vi "Powerlawfit_Ranjani.vi"() -> ()   [LabVIEW 2020]
uses:
  <vilib>/Analysis/NI_AALPro.lvlib
panel:
  in  "parameter bounds":T1={"amp min"=-inf, "amp max"=inf, "power min"=-inf, "power max"=inf, "offset min"=-0.0001, "offset max"=0.0001}
  out "residue":dbl=1.2236868285246925e-12
  out "amplitude":dbl=1.9889547263019e-06
  out "Fitoffset":dbl=1.9090068470777766e-05
  out "power":dbl=2.2722781909445917
  in  "Tab Control":enum32{"Drag R and 4T R", " Line cut"}(tab)=enum." Line cut"
  in  "Input figure":cluster{dbl[], dbl[]}[](graph)
  out "Mean vs Curve":cluster{dbl[], dbl[]}(graph)
  in  "Group #":i32=40
  out "Power vs Cursorx":cluster{dbl[], dbl[]}(graph)
  out "Waveform Chart":T2(graph)={"Cursor.Cursor Y"=8.581818181818182, "Cursor.Cursor X"=0.002007000000000002}
  in  "Drag V from V2":dbl[][](graph)=array1800x28[50400 elements]
  out "Vcut":cluster{dbl[], "Best Power Fit":dbl[]}[](graph)=[{[1.2, 1.3, 1.4, 1.5, 1.6, 1.7, 1.8, 1.9, 2.0, 2.1, 2.2, 2.3, 2.4000000000000004, 2.5, 2.6, 2.7, 2.8, 2.9000000000000004, 3.0, 3.1, 3.2, 3.3, 3.4000000000000004, 3.5, 3.6000000000000005, 3.7, 3.8, 3.9000000000000004], "Best Power Fit"=[2.015930672170834e-05, 2.0795129581608732e-05, 2.1820384012533006e-05, 2.280280711999687e-05, 2.3946763648175132e-05, 2.5134933511751197e-05, 2.6181392071272518e-05, 2.7929617110195616e-05, 2.9262532189874433e-05, 3.054493768019253e-05, 3.19082066212991e-05, 3.363555114887107e-05, 3.4788814987151014e-05, 3.678953448119711e-05, 3.780095419235919e-05, 3.970849457050918e-05, 4.096530292161228e-05, 4.254818023165695e-05, 4.432108587672819e-05, 4.546588214924085e-05, 4.748056918344682e-05, 4.8810664172975e-05, 5.080883573646553e-05, 5.2979622295762476e-05, 5.479300628442206e-05, 5.697505105039216e-05, 5.889263564225451e-05, 6.207291546365798e-05]}, {[1.2, 1.3, 1.4, 1.5, 1.6, 1.7, 1.8, 1.9, 2.0, 2.1, 2.2, 2.3, 2.4000000000000004, 2.5, 2.6, 2.7, 2.8, 2.9000000000000004, 3.0, 3.1, 3.2, 3.3, 3.4000000000000004, 3.5, 3.6000000000000005, 3.7, 3.8, 3.9000000000000004], "Best Power Fit"=[2.209993138662107e-05, 2.2700306960527264e-05, 2.3362434430446028e-05, 2.408757333096512e-05, 2.4876919233962166e-05, 2.573161096568624e-05, 2.6652736615764704e-05, 2.76413385987508e-05, 2.8698417961369154e-05, 2.9824938081228762e-05, 3.1021827868784444e-05, 3.22899845594946e-05, 3.3630276164677404e-05, 3.504354363566098e-05, 3.653060278519871e-05, 3.809224600190149e-05, 3.972924378701247e-05, 4.144234613777122e-05, 4.323228379756374e-05, 4.509976938979739e-05, 4.704549844979653e-05, 4.907015036685682e-05, 5.1174389246819735e-05, 5.33588647040583e-05, 5.562421259054056e-05, 5.797105566861031e-05, 6.040000423326106e-05, 6.291165668894683e-05]}]
  out "Idrive":cluster{dbl[], dbl[]}[](graph)=[{[-0.009243, -0.009233, -0.009223, -0.009212999999999999, -0.009203, -0.009193, -0.009183, -0.009172999999999999, -0.009163, -0.009153, -0.009143, -0.009132999999999999, -0.009123, -0.009113, -0.009103, -0.009092999999999999, -0.009082999999999999, -0.009073, -0.009063, -0.009053, -0.009042999999999999, -0.009033, -0.009023, -0.009013, -0.009002999999999999, -0.008993, -0.008983, -0.008973], []}]
  out "Residue of T vs Cursorx":cluster{dbl[], dbl[]}(graph)
  in  "stop":bool
  # "Vsd  = 0V, a = 3.3\nVsd  = -500uV, a = 3.1\nVsd  = -1mV, a = 2.67\nVsd  = 500uV, a = 3.04\nVsd  = 1mV, a = 2.6"
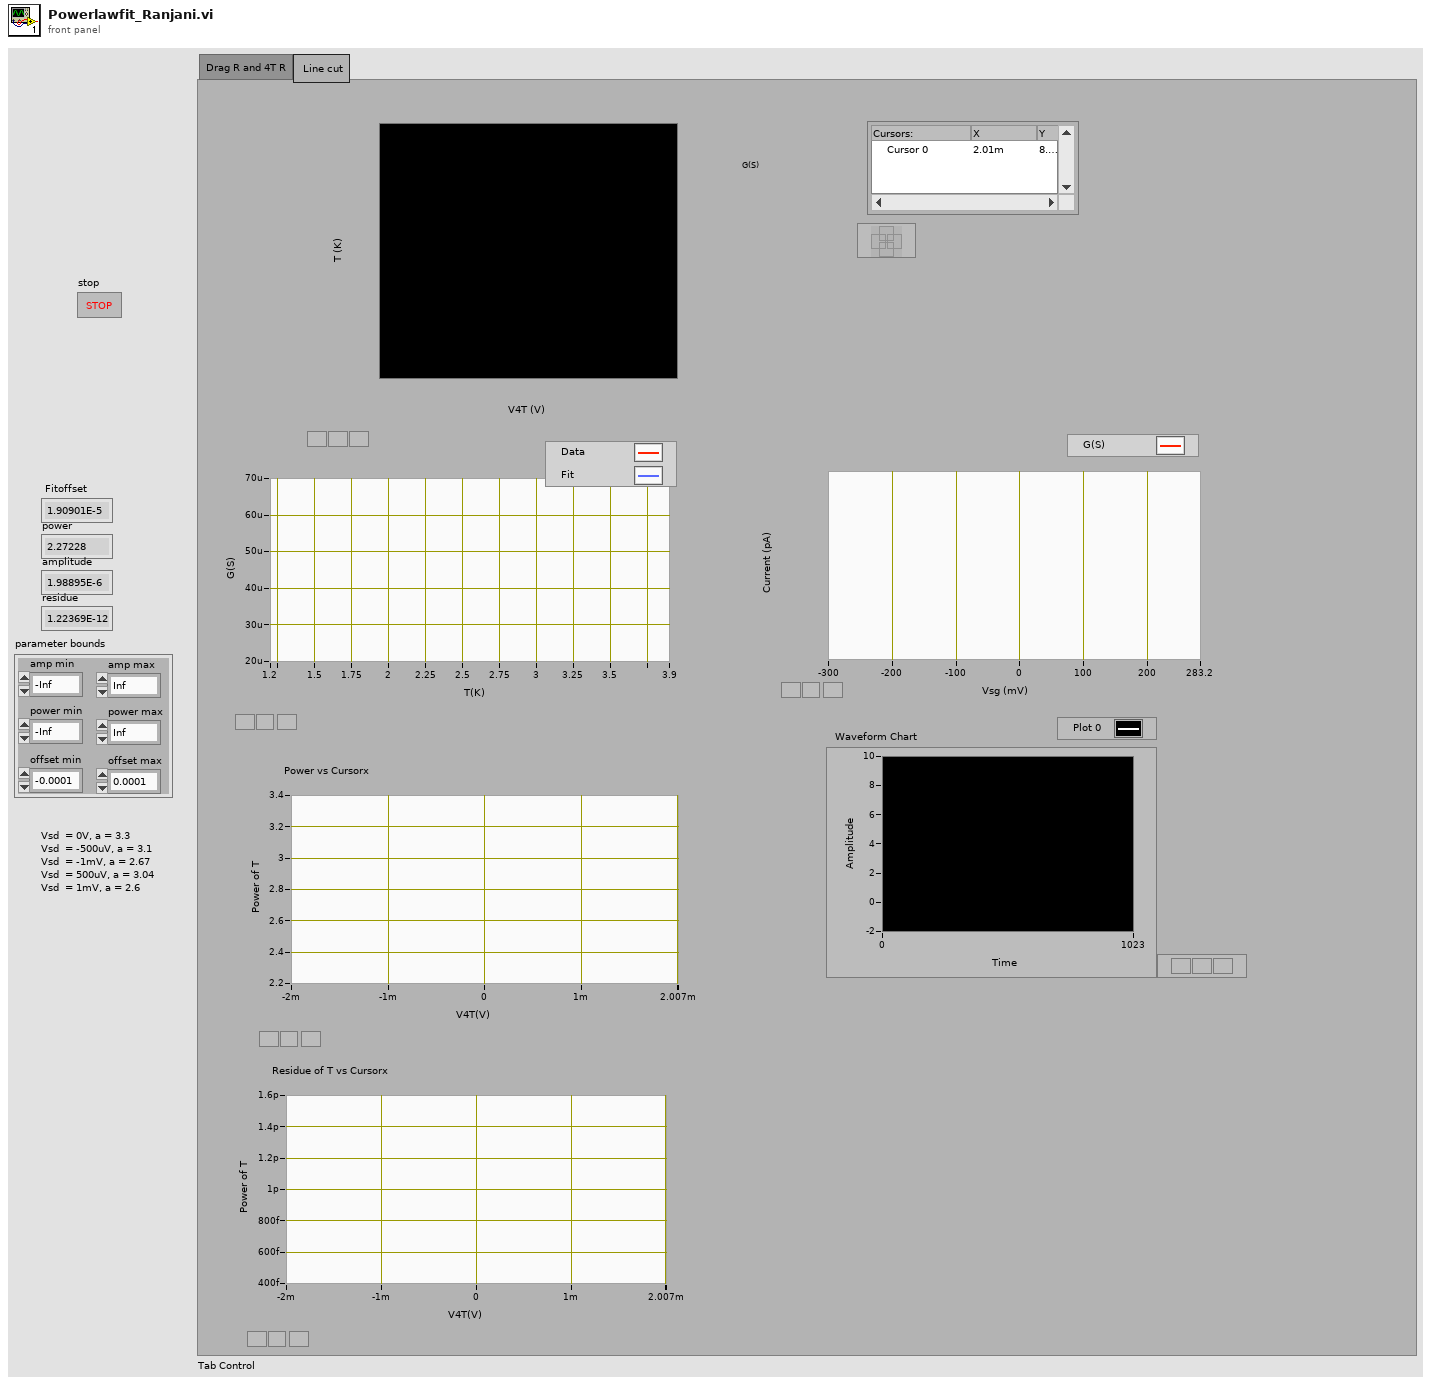
[diagram p1: front panel]
types:
  T1 = cluster{"amp min":dbl, "amp max":dbl, "power min":dbl, "power max":dbl, "offset min":dbl, "offset max":dbl}
  T2 = cluster{"Cursor.Cursor Y":dbl, "Cursor.Cursor X":dbl}
  T3 = typedef "LVOffsetAndMultiplierTypeDef.ctl" = cluster{"Offset":dbl, "Multiplier":dbl}
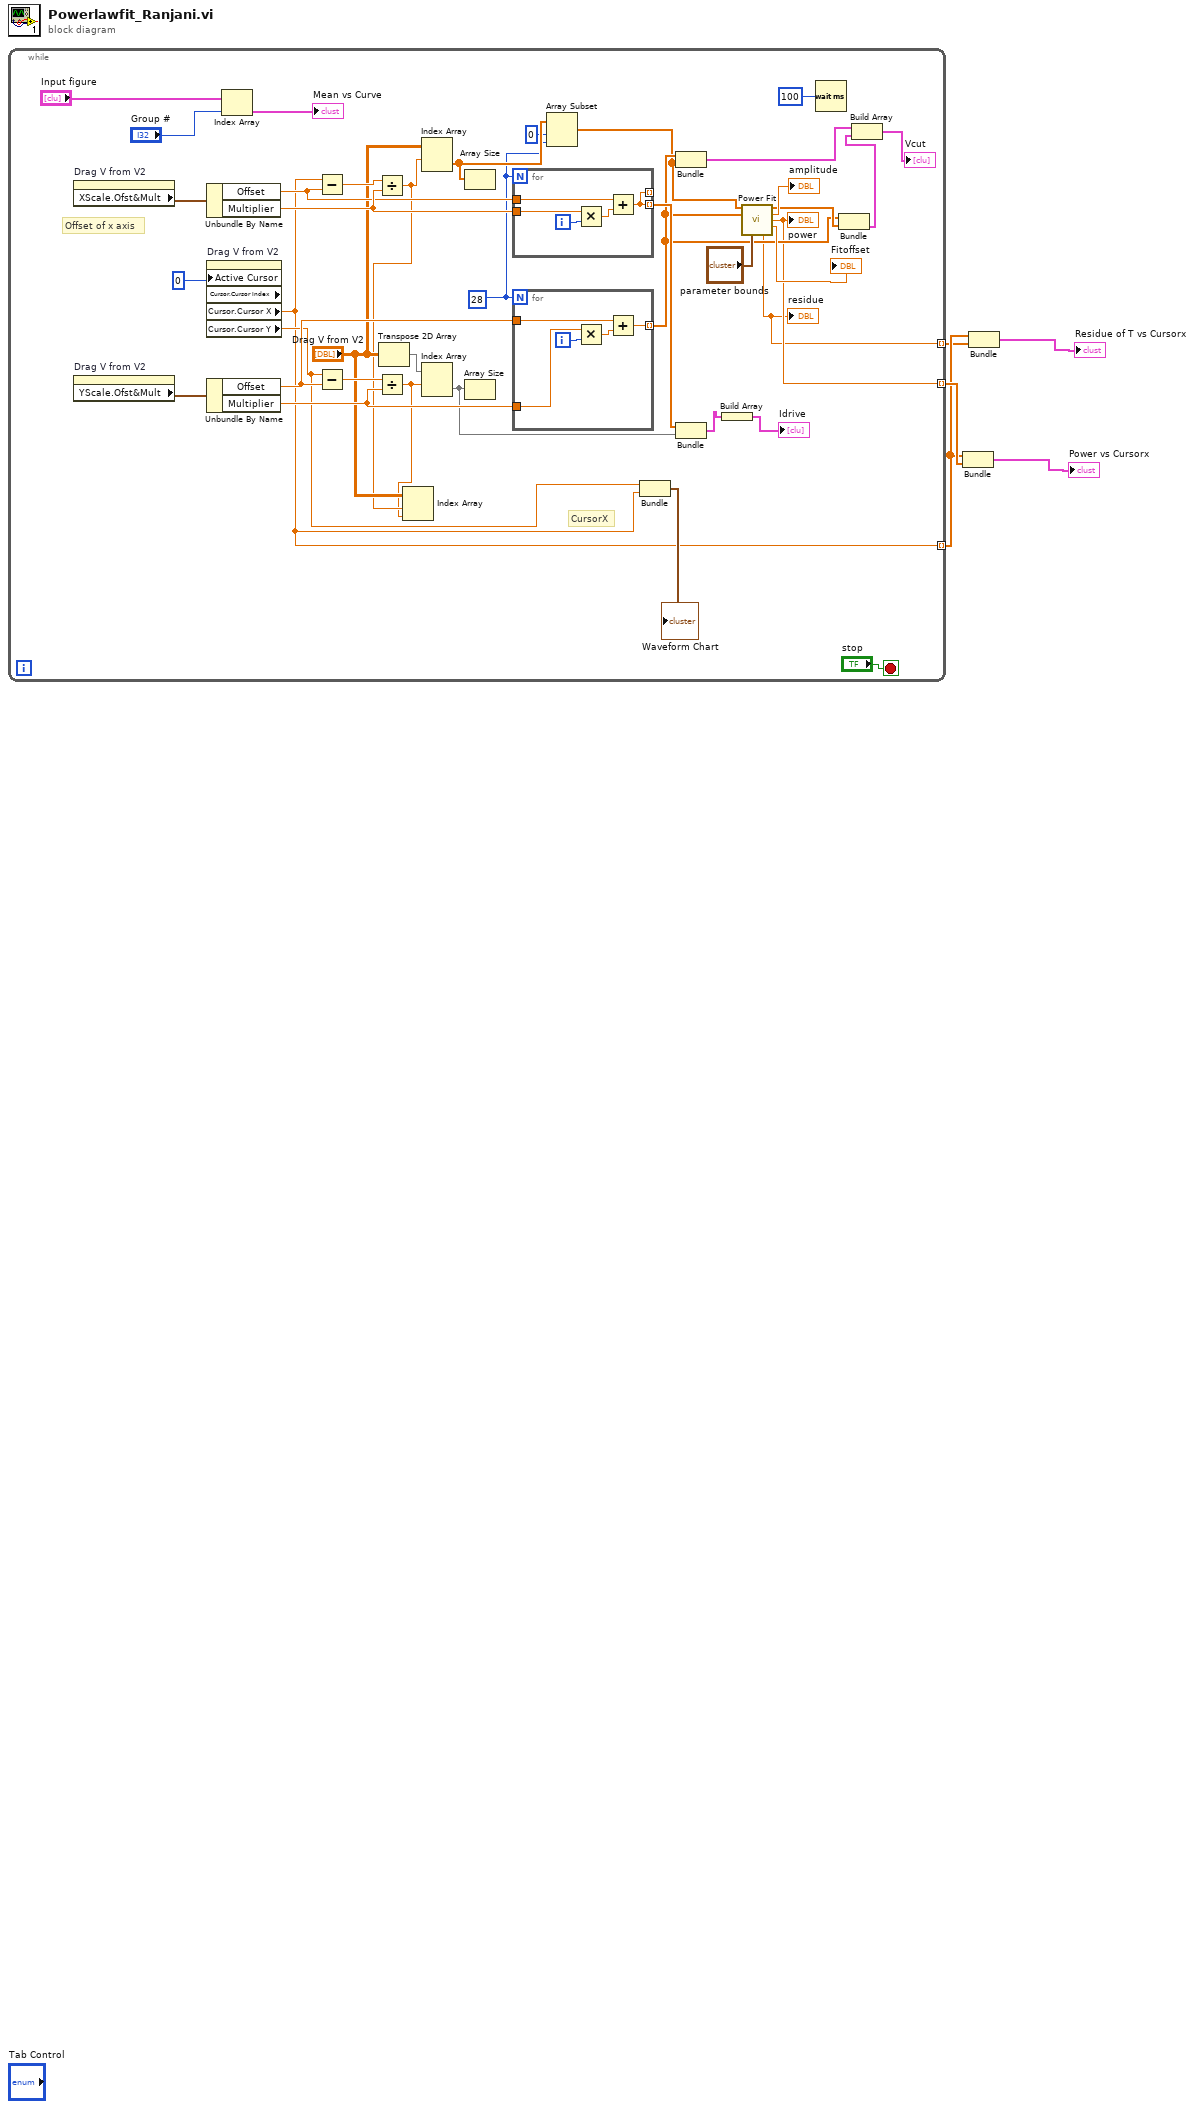
[diagram p0: block diagram]
diagram:
  n1 = while {
    tunnel: [w22] -> w2 mode=indexing
    tunnel: [w11] -> w4 mode=indexing
    tunnel: [w10] -> w1 mode=indexing
    stop <- "stop" stop-if-true
    w6 = 28
    # "CursorX"
    # "Offset of x axis"
    n2 = property on="Drag V from V2" class="IntGraph (strict)"() -> ("XScale.Ofst&Mult"=w37:T3)  [unwired: 2 in, 2 out]
    n3 = property on="Drag V from V2" class="IntGraph (strict)"() -> ("YScale.Ofst&Mult"=w39:T3)  [unwired: 2 in, 2 out]
    n4 = Unbundle By Name(w37) -> ("Offset"=w31:dbl, "Multiplier"=w32:dbl)
    n5 = property on="Drag V from V2" class="IntGraph (strict)" props=["Active Cursor", "Cursor", "Cursor Index", "Cursor", "Cursor X", "Cursor", "Cursor Y"]("Active Cursor"=u32 0) -> ("Cursor.Cursor X"=w22:dbl, "Cursor.Cursor Y"=w23:dbl)  [unwired: 2 in, 3 out]
    n6 = Unbundle By Name(w39) -> ("Offset"=w34:dbl, "Multiplier"=w35:dbl)
    n7 = Index Array(array="Input figure", index="Group #") -> (element=→"Mean vs Curve":cluster{dbl[], dbl[]})
    n8 = Subtract(x=w22, y=w31) -> (x-y=w36:dbl)
    n9 = Subtract(x=w23, y=w34) -> (x-y=w38:dbl)
    n10 = Divide(x=w36, y=w32) -> (x/y=w27:dbl)
    n11 = Divide(x=w38, y=w35) -> (x/y=w26:dbl)
    n12 = Transpose 2D Array(2D array="Drag V from V2") -> (transposed array=w41:dbl[][])
    n13 = Index Array(array="Drag V from V2", index (row)=w27, index (col)=w26) -> ()  [unwired: 1 out]
    n14 = Index Array(array="Drag V from V2", index (row)=w27) -> (element=w9:dbl[])  [unwired: 1 in]
    n15 = Index Array(array=w41, index (row)=w26) -> (element=w33:dbl[])  [unwired: 1 in]
    n16 = Array Size(array=w9) -> ()  [unwired: 1 out]
    n17 = Array Size(array=w33) -> ()  [unwired: 1 out]
    n18 = for {
      N: w6 -> [_]
      tunnel: w32 -> [w48]
      tunnel: w31 -> [w46]
      tunnel: [w45] -> _ mode=indexing
      tunnel: [w45] -> w30 mode=indexing
      i -> [w49]
      n19 = Multiply(x=w48, y=w49) -> (x*y=w47:dbl)
      n20 = Add(x=w46, y=w47) -> (x+y=w45:dbl)
    }
    n21 = for {
      N: w6 -> [_]
      tunnel: w35 -> [w53]
      tunnel: w34 -> [w51]
      tunnel: [w50] -> w15 mode=indexing
      i -> [w54]
      n22 = Multiply(x=w53, y=w54) -> (x*y=w52:dbl)
      n23 = Add(x=w51, y=w52) -> (x+y=w50:dbl)
    }
    n24 = Array Subset(array=w9, index=0, length=w6) -> (w8:dbl[])
    n25 = Bundle("Cursor.Cursor Y"=w23, "Cursor.Cursor X"=w22) -> (→"Waveform Chart":T2)  [unwired: 1 in]
    n26 = Bundle(w15, w8) -> (w13:cluster{dbl[], dbl[]})  [unwired: 1 in]
    n27 = Bundle(w30, w33) -> (w21:cluster{dbl[], dbl[]})  [unwired: 1 in]
    n28 = Build Array(w21) -> (→"Idrive":cluster{dbl[], dbl[]}[])
    n29 = call <vilib>:"Power Fit.vi"("Y"=w8, "X"=w15, "parameter bounds"="parameter bounds") -> ("Best Power Fit"=w16:dbl[], "amplitude"=→"amplitude":dbl, "power"=w11:dbl, "offset"=→"Fitoffset":dbl, "residue"=w10:dbl)  [unwired: 7 in, 1 out]
    "power" <- w11
    "residue" <- w10
    n30 = Wait (ms)(milliseconds to wait=u32 100) -> ()  [unwired: 1 out]
    n31 = Bundle(w15, "Best Power Fit"=w16) -> (w14:cluster{dbl[], "Best Power Fit":dbl[]})  [unwired: 1 in]
    n32 = Build Array(w13, w14) -> (→"Vcut":cluster{dbl[], "Best Power Fit":dbl[]}[])
  }
  n33 = Bundle(w2, w4) -> (→"Power vs Cursorx":cluster{dbl[], dbl[]})  [unwired: 1 in]
  n34 = Bundle(w2, w1) -> (→"Residue of T vs Cursorx":cluster{dbl[], dbl[]})  [unwired: 1 in]
